vi "data_manipulation_MLP2.vi"(11 "Array in":fxp<+/-,32,16>[](array[numeric])=[0.0, 0.0, 0.0, 0.0, 0.0, 0.0, 0.0, 0.0, 0.0, 0.0, 0.0, 0.0]) -> (3 "Array out":fxp<+/-,64,35>[](array[numeric]))   [LabVIEW 2020]
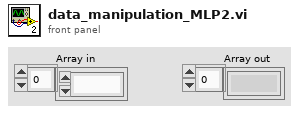
[diagram p1: front panel]
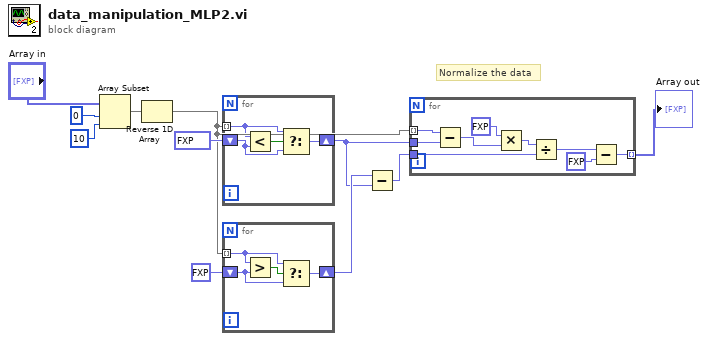
[diagram p0: block diagram]
diagram:
  # "Normalize the data"
  n1 = Array Subset(array="Array in", index=0, length=10) -> (w2:fxp<+/-,32,16>[])
  n2 = Reverse 1D Array(array=w2) -> (reversed array=w1:fxp<+/-,32,16>[])
  n3 = for {
    tunnel: w1 -> [w13] mode=indexing
    shift-right: [w15] -> w4
    shift-left: fxp<+,11,15> 30000.0 -> [w12]
    n4 = Less?(x=w13, y=w12) -> (x < y?=w14:bool)
    n5 = Select(t=w13, s=w14, f=w12) -> (s? t:f=w15:fxp<+/-,32,16>)
  }
  n6 = for {
    tunnel: w1 -> [w18] mode=indexing
    shift-right: [w16] -> w5
    shift-left: fxp<+,1,1> 0.0 -> [w17]
    n7 = Greater?(x=w18, y=w17) -> (0:w19:bool)
    n8 = Select(t=w18, s=w19, f=w17) -> (s? t:f=w16:fxp<+/-,32,16>)
  }
  n9 = Subtract(x=w5, y=w4) -> (x-y=w3:fxp<+/-,33,17>)
  n10 = for {
    tunnel: w1 -> [w28] mode=indexing
    tunnel: [w22] -> w11 mode=indexing
    tunnel: w4 -> [w27]
    tunnel: w3 -> [w24]
    n11 = Subtract(x=w28, y=w27) -> (x-y=w26:fxp<+/-,33,17>)
    n12 = Multiply(x=fxp<+,1,2> 2.0, y=w26) -> (x*y=w25:fxp<+/-,33,18>)
    n13 = Divide(x=w25, y=w24) -> (x/y=w23:fxp<+/-,64,34>)
    n14 = Subtract(x=w23, y=fxp<+,1,1> 1.0) -> (x-y=w22:fxp<+/-,64,35>)
  }
  "Array out" <- w11
